vi "Calculate Message Timeout.vi"(9 "Result Parsing Timeout":i32, 10 "Message Timeout":i32, 11 "Module Timeout":i32) -> (3 "Calculated Timeout":i32)   [LabVIEW 2017, in "SSH.lvlib"]
uses:
  SSH.lvlib
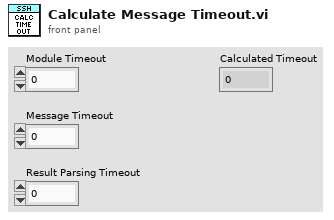
[diagram p1: front panel]
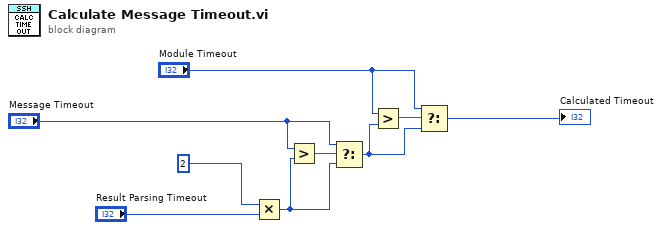
[diagram p0: block diagram]
diagram:
  n1 = Multiply(x=2, y="Result Parsing Timeout") -> (x*y=w1:i32)
  n2 = Greater?(x="Message Timeout", y=w1) -> (0:w3:bool)
  n3 = Select(t="Message Timeout", s=w3, f=w1) -> (s? t:f=w7:i32)
  n4 = Greater?(x="Module Timeout", y=w7) -> (0:w6:bool)
  n5 = Select(t="Module Timeout", s=w6, f=w7) -> (s? t:f=→"Calculated Timeout":i32)
